vi "Euclidean_dist.vi"(10 "y":sgl[][](array[numeric]), 11 "x":sgl[][](array[numeric])) -> (3 "distances":sgl[][](array[numeric]))   [LabVIEW 2020]
uses:
  <vilib>/addons/Multicore Analysis and Sparse Matrix/BLAS/_blas/Transpose.ctl
  <vilib>/addons/Multicore Analysis and Sparse Matrix/BLAS/gemv - General Matrix-Vector Product.vi
  <vilib>/addons/Multicore Analysis and Sparse Matrix/BLAS/_blas/sgemv - General Matrix-Vector Product (SGL).vi
  <vilib>/addons/Multicore Analysis and Sparse Matrix/BLAS/_blas/sgemm - General Matrix-Matrix Product (SGL).vi
  <vilib>/addons/Multicore Analysis and Sparse Matrix/BLAS/NI_MASM_BLAS.lvlib
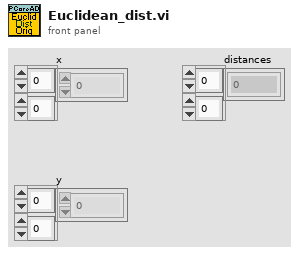
[diagram p1: front panel]
types:
  T1 = typedef "NI_MASM_BLAS.lvlib/Transpose.ctl" = i32
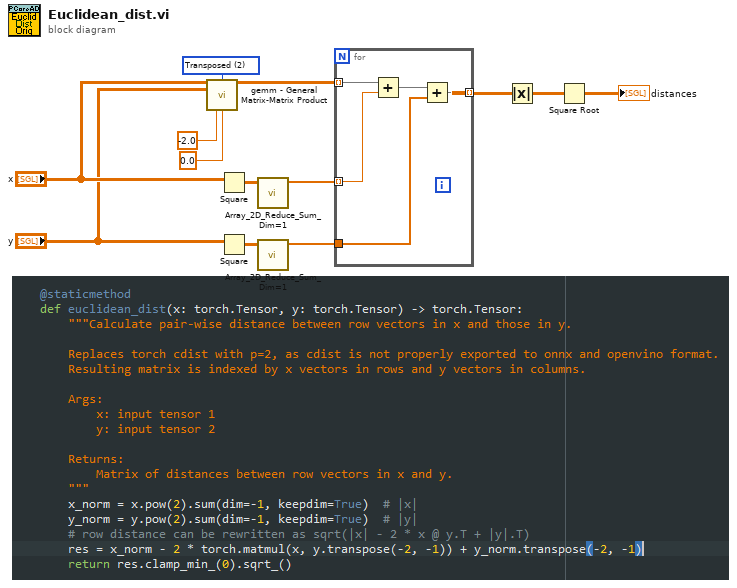
[diagram p0: block diagram]
diagram:
  w13 = T1 2 items=["Direct", "Conjugated & Transposed", "Transposed"] ("operation B")
  n1 = call-poly <vilib>:"gemm - General Matrix-Matrix Product.vi"("A"="x", "operation B"=w13, "B"="y", "alpha"=sgl -2.0, "beta"=sgl 0.0) -> ("sgemm"=w9:sgl[][])  [unwired: 9 in, 1 out]
  n2 = Square(x="x") -> (x^2=w4:sgl[][])
  n3 = Square(x="y") -> (x^2=w3:sgl[][])
  n4 = call "Array_2D_Reduce_Sum_Dim=1.vi"("x"=w4) -> ("x out"=w2:sgl[])  [unwired: 10 in]
  n5 = call "Array_2D_Reduce_Sum_Dim=1.vi"("x"=w3) -> ("x out"=w1:sgl[])  [unwired: 10 in]
  n6 = for {
    tunnel: w9 -> [w17] mode=indexing
    tunnel: w2 -> [w18] mode=indexing
    tunnel: [w15] -> w7 mode=indexing
    tunnel: w1 -> [w14]
    n7 = Add(x=w17, y=w18) -> (x+y=w16:sgl[])
    n8 = Add(x=w16, y=w14) -> (x+y=w15:sgl[])
  }
  n9 = Absolute Value(x=w7) -> (abs(x)=w6:sgl[][])
  n10 = Square Root(x=w6) -> (sqrt(x)=→"distances":sgl[][])
